vi "GDSString_PlaceHolderText.vi"(6 "BooleanUserEventToStopPlaceHolderVI":refnum<user-event>, 7 "PlaceholderText":string, 8 "error in (no error)":errorcluster, 9 "PlaceholderTextFont(Grey,Italic)":T1={"Font Name"="", "Size"=0, "Bold"=FALSE, "Italic"=TRUE, "Underline"=FALSE, "Strikeout"=FALSE, "Color"=10329501}, 10 "NormalTextFont(Black)":T1, 11 "PlaceholderStringRef":refnum<vi>) -> (0 "error out":errorcluster)   [LabVIEW 2020]
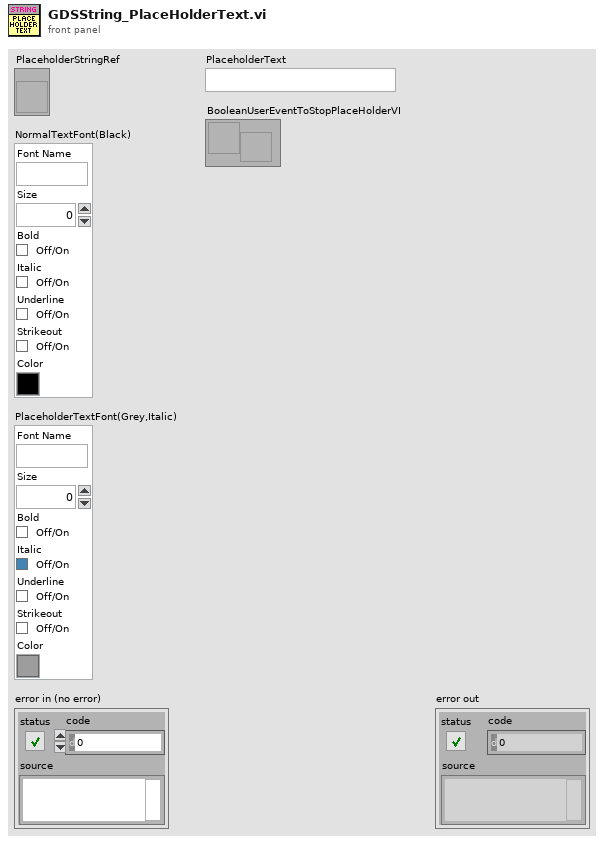
[diagram p1: front panel]
types:
  T1 = cluster{"Font Name":string, "Size":u16, "Bold":bool, "Italic":bool, "Underline":bool, "Strikeout":bool, "Color":u32}
  T2 = typedef "LVFontTypeDef.ctl" = cluster{"Font Name":string, "Size":u16, "Bold":bool, "Italic":bool, "Underline":bool, "Strikeout":bool, "Color":u32}
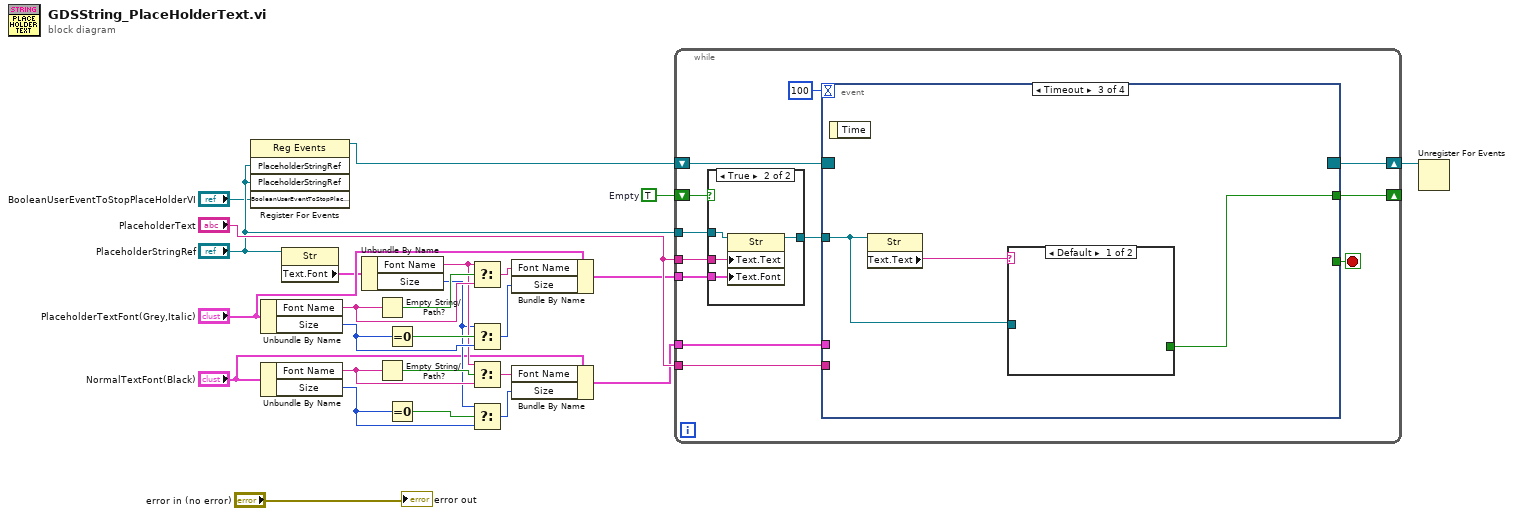
[diagram p0: block diagram]
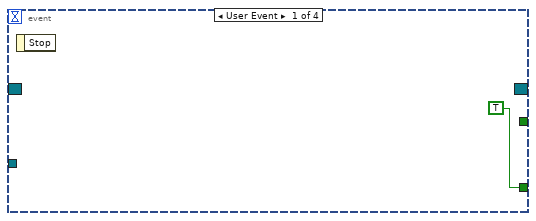
[diagram p3: hidden frame]
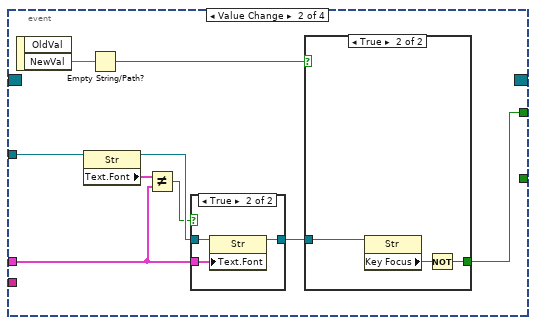
[diagram p4: hidden frame]
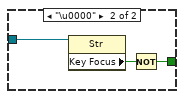
[diagram p7: hidden frame]
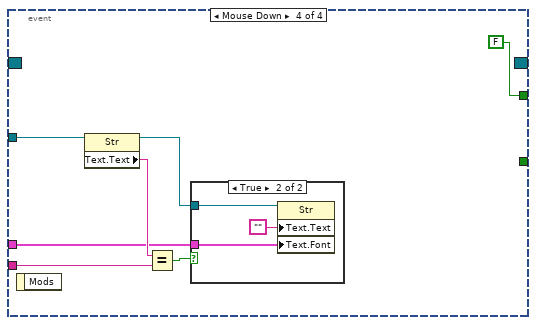
[diagram p8: hidden frame]
diagram:
  w23 = TRUE  # Empty
  n1 = register-events("PlaceholderStringRef", "PlaceholderStringRef", "BooleanUserEventToStopPlaceHolderVI") -> (reference out=w26:refnum<event-registration>)  [unwired: 2 in, 1 out]
  n2 = Unbundle By Name("PlaceholderTextFont(Grey,Italic)") -> ("Font Name"=w19:string, "Size"=w14:u16)
  n3 = Unbundle By Name("NormalTextFont(Black)") -> ("Font Name"=w9:string, "Size"=w13:u16)
  n4 = property class="Str"(reference="PlaceholderStringRef") -> ("Text.Font"=w21:T2)  [unwired: 1 in, 2 out]
  n5 = Unbundle By Name(w21) -> ("Font Name"=w7:string, "Size"=w6:u16)
  n6 = Empty String/Path?(string/path=w19) -> (empty?=w20:bool)
  n7 = Empty String/Path?(string/path=w9) -> (empty?=w8:bool)
  n8 = Equal To 0?(x=w14) -> (x = 0?=w16:bool)
  n9 = Equal To 0?(x=w13) -> (x = 0?=w11:bool)
  n10 = Select(t=w7, s=w20, f=w19) -> (s? t:f=w17:string)
  n11 = Select(t=w6, s=w16, f=w14) -> (s? t:f=w15:u16)
  n12 = Select(t=w7, s=w8, f=w9) -> (s? t:f=w10:string)
  n13 = Select(t=w6, s=w11, f=w13) -> (s? t:f=w12:u16)
  n14 = Bundle By Name(cluster="PlaceholderTextFont(Grey,Italic)", "Font Name"=w17, "Size"=w15) -> (w18:T1)
  n15 = Bundle By Name(cluster="NormalTextFont(Black)", "Font Name"=w10, "Size"=w12) -> (w4:T1)
  n16 = while {
    shift-right: [w37] -> w25
    shift-left: w26 -> [w38]
    tunnel: "PlaceholderText" -> [w36]
    tunnel: "PlaceholderStringRef" -> [w35]
    tunnel: "PlaceholderText" -> [w32]
    shift-right: [w30] -> _
    shift-left: w23 -> [w31]
    tunnel: w18 -> [w29]
    tunnel: w4 -> [w28]
    stop <- w34 stop-if-true
    n17 = case shown="True" w31 {
      tunnel: w36 -> [_ w43]
      tunnel: w35 -> [w39 w42]
      tunnel: [w39 w41] -> w33
      tunnel: w29 -> [_ w40]
      frame False {
      }
      frame True {
        n18 = property class="Str"(reference=w42, "Text.Text"=w43, "Text.Font"=w40) -> (reference out=w41:refnum<vi>)  [unwired: 1 in, 1 out]
      }
    }
    n19 = event shown="[2] Timeout" {
      selector: w38 -> [_ _ _ _]
      dyn-events: [_ _ _ _] -> w37
      timeout: 100 -> [_ _ _ _]
      tunnel: [TRUE _ _ _] -> w34
      tunnel: w33 -> [_ w50 w62 w73]
      tunnel: w32 -> [_ _ _ w71]
      tunnel: [_ w51 w61 FALSE] -> w30
      tunnel: w28 -> [_ w46 _ w67]
      event User Event {
        n20 = event-data() -> ()  [unwired: 1 in, 1 out]
      }
      event Value Change {
        n21 = event-data() -> ("NewVal"=w53:string)  [unwired: 1 in, 1 out]
        n22 = property class="Str"(reference=w50) -> (reference out=w48:refnum<vi>, "Text.Font"=w49:T2)  [unwired: 1 in, 1 out]
        n23 = Empty String/Path?(string/path=w53) -> (empty?=w52:bool)
        n24 = Not Equal?(x=w49, y=w46) -> (x != y?=w45:bool)
        n25 = case shown="True" w45 {
          tunnel: w48 -> [w54 w57]
          tunnel: [w54 w56] -> w47
          tunnel: w46 -> [_ w55]
          frame False {
          }
          frame True {
            n26 = property class="Str"(reference=w57, "Text.Font"=w55) -> (reference out=w56:refnum<vi>)  [unwired: 1 in, 1 out]
          }
        }
        n27 = case shown="True" w52 {
          tunnel: w47 -> [_ w60]
          tunnel: [_ w58] -> w51
          frame False {
          }
          frame True {
            n28 = property class="Str"(reference=w60) -> ("Key Focus"=w59:bool)  [unwired: 1 in, 2 out]
            n29 = Not(x=w59) -> (.not. x?=w58:bool)
          }
        }
      }
      event Timeout {
        n30 = event-data() -> ()  [unwired: 1 in, 1 out]
        n31 = property class="Str"(reference=w62) -> ("Text.Text"=w63:string)  [unwired: 1 in, 2 out]
        n32 = case shown="Default" w63 {
          tunnel: w62 -> [_ w66]
          tunnel: [_ w64] -> w61
          frame Default {
          }
          frame "\u0000" {
            n33 = property class="Str"(reference=w66) -> ("Key Focus"=w65:bool)  [unwired: 1 in, 2 out]
            n34 = Not(x=w65) -> (.not. x?=w64:bool)
          }
        }
      }
      event Mouse Down {
        n35 = event-data() -> ()  [unwired: 1 in, 1 out]
        n36 = property class="Str"(reference=w73) -> (reference out=w70:refnum<vi>, "Text.Text"=w72:string)  [unwired: 1 in, 1 out]
        n37 = Equal?(x=w72, y=w71) -> (x = y?=w69:bool)
        n38 = case shown="True" w69 {
          tunnel: w70 -> [_ w76]
          tunnel: w67 -> [_ w74]
          frame False {
          }
          frame True {
            n39 = property class="Str"(reference=w76, "Text.Text"="", "Text.Font"=w74) -> ()  [unwired: 1 in, 2 out]
          }
        }
      }
    }
  }
  n40 = Unregister For Events(event registration refnum=w25) -> ()  [unwired: 1 in, 1 out]
  "error out" <- "error in (no error)"
